vi "习4.7.vi"() -> ()   [LabVIEW 2017]
panel:
  out "数值":i32
  out "猜测次数":i32
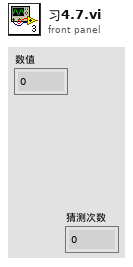
[diagram p1: front panel]
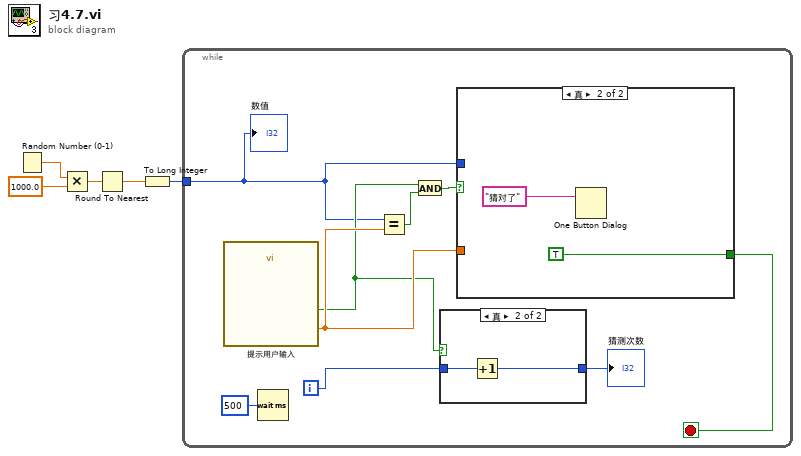
[diagram p0: block diagram]
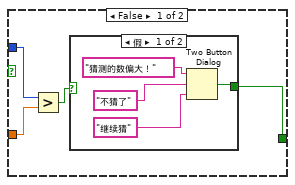
[diagram p3: hidden frame]
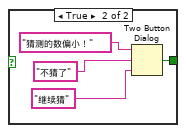
[diagram p4: hidden frame]
diagram:
  n1 = Random Number (0-1)() -> (number: 0 to 1=w5:dbl)
  n2 = Multiply(x=w5, y=1000.0) -> (x*y=w3:dbl)
  n3 = Round To Nearest(number=w3) -> (nearest integer value=w2:dbl)
  n4 = To Long Integer(number=w2) -> (32bit integer=w1:i32)
  n5 = while {
    tunnel: w1 -> [w6]
    i -> [w10]
    stop <- w8 stop-if-true
    n6 = call "提示用户输入"() -> ("请在1-1000猜"=w12:dbl, "确定"=w11:bool)  [unwired: 17 in, 1 out]
    n7 = Wait (ms)(milliseconds to wait=u32 500 ("等待时间（毫秒）")) -> ()  [unwired: 1 out]
    n8 = Equal?(x=w6, y=w12) -> (x = y?=w14:bool)
    n9 = And(x=w11, y=w14) -> (x .and. y?=w13:bool)
    n10 = case shown="真" w11 {
      tunnel: w10 -> [w15 w17]
      tunnel: [w15 w16] -> w9
      frame False {
      }
      frame True {
        n11 = Increment(x=w17) -> (x+1=w16:i32)
      }
    }
    "猜测次数" <- w9
    n12 = case shown="真" w13 {
      tunnel: w6 -> [w20 _]
      tunnel: w12 -> [w19 _]
      tunnel: [w18 TRUE] -> w8
      frame False {
        n13 = Greater?(x=w20, y=w19) -> (0:w21:bool)
        n14 = case shown="假" w21 {
          tunnel: [w25 w26] -> w18
          frame False {
            n15 = Two Button Dialog(message="猜测的数偏大！", 1:"继续猜", 2:"不猜了") -> (T button?=w25:bool)
          }
          frame True {
            n16 = Two Button Dialog(message="猜测的数偏小！", 1:"继续猜", 2:"不猜了") -> (T button?=w26:bool)
          }
        }
      }
      frame True {
        n17 = One Button Dialog(message="猜对了") -> ()  [unwired: 1 in, 1 out]
      }
    }
    "数值" <- w6
  }
